vi "External Shutdown.vi"(8 "error in (no error)":errorcluster, 11 "Accelerometer in":refnum<class "Accelerometer.lvclass">) -> (0 "error out":errorcluster, 3 "Accelerometer out":refnum<class "Accelerometer.lvclass">)   [LabVIEW 2020, in "Accelerometer.lvlib" / "Accelerometer.lvclass"]
uses:
  Accelerometer.lvclass
  Accelerometer.lvclass/Accelerometer.ctl
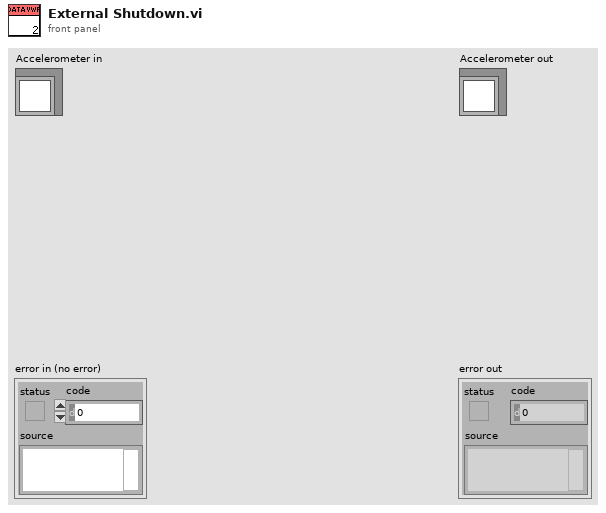
[diagram p1: front panel]
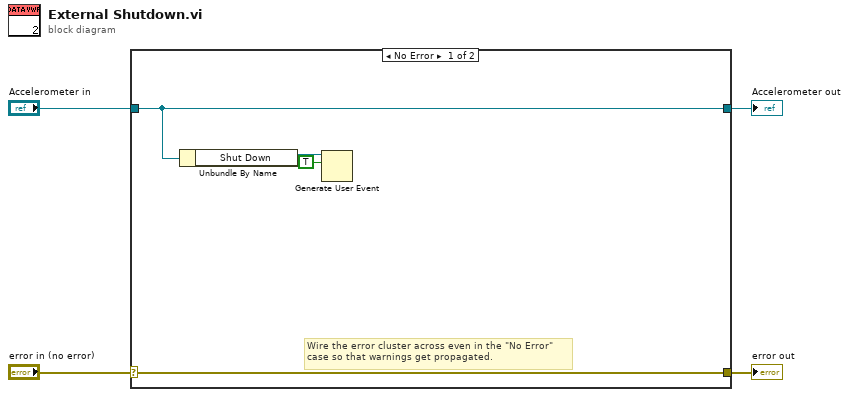
[diagram p0: block diagram]
diagram:
  n1 = case shown="No Error" "error in (no error)" {
    selector: "error in (no error)" -> [w8 w10]
    tunnel: [w8 w10] -> w3
    tunnel: [w7 w9] -> w1
    tunnel: "Accelerometer in" -> [w7 w9]
    frame No Error {
      # "Wire the error cluster across even in the \"No Error\"\ncase so that warnings get propagated."
      n2 = Unbundle By Name(w7) -> ("Shut Down"=w6:refnum<user-event>)
      n3 = Generate User Event(user event=w6, event data cluster=TRUE ("event data")) -> ()  [unwired: 2 in, 2 out]
    }
    frame Error {
    }
  }
  "error out" <- w3
  "Accelerometer out" <- w1
